vi "UnscentedKalmanFilter_SetXHat_Single.vi"(9 "xHat Value":dbl, 10 "Row":i32, 11 "in UnscentedKalmanFiilter":T1) -> (3 "out UnscentedKalmanFiilter":T1)   [LabVIEW 2019, in "Trajectory_Library.lvlib"]
doc: "Creates a new LINEAR SYSTEM data cluster with the specified values. \n\n\nInputs: \n - XXX -- XXX.\n\nOutputs:\n - XXX -- XXX."
uses:
  Trajectory_Library.lvlib
  <vilib>/Analysis/Matrix/Datatypes/RealMatrix.ctl
  <vilib>/Analysis/Matrix/NI_Matrix.lvlib
  MERWE_SCALED_SIGMA_PTS.ctl
  UNSCENTED_KALMAN_FILTER.ctl
  BiFun_Matrix_FUNC_TYPE.ctl
panel:
  # "State Estimate <Statess,1>"
  # "<States, States>"
  # "<States, ?>"
  # "<Statess,  States>"
  # "<Outputs, Outputs>"
  # "<?, 1>"
  # "<?, 1>"
  # "State Estimate <Statess,1>"
  # "<States, States>"
  # "<States, ?>"
  # "<Statess,  States>"
  # "<Outputs, Outputs>"
  # "<?, 1>"
  # "<?, 1>"
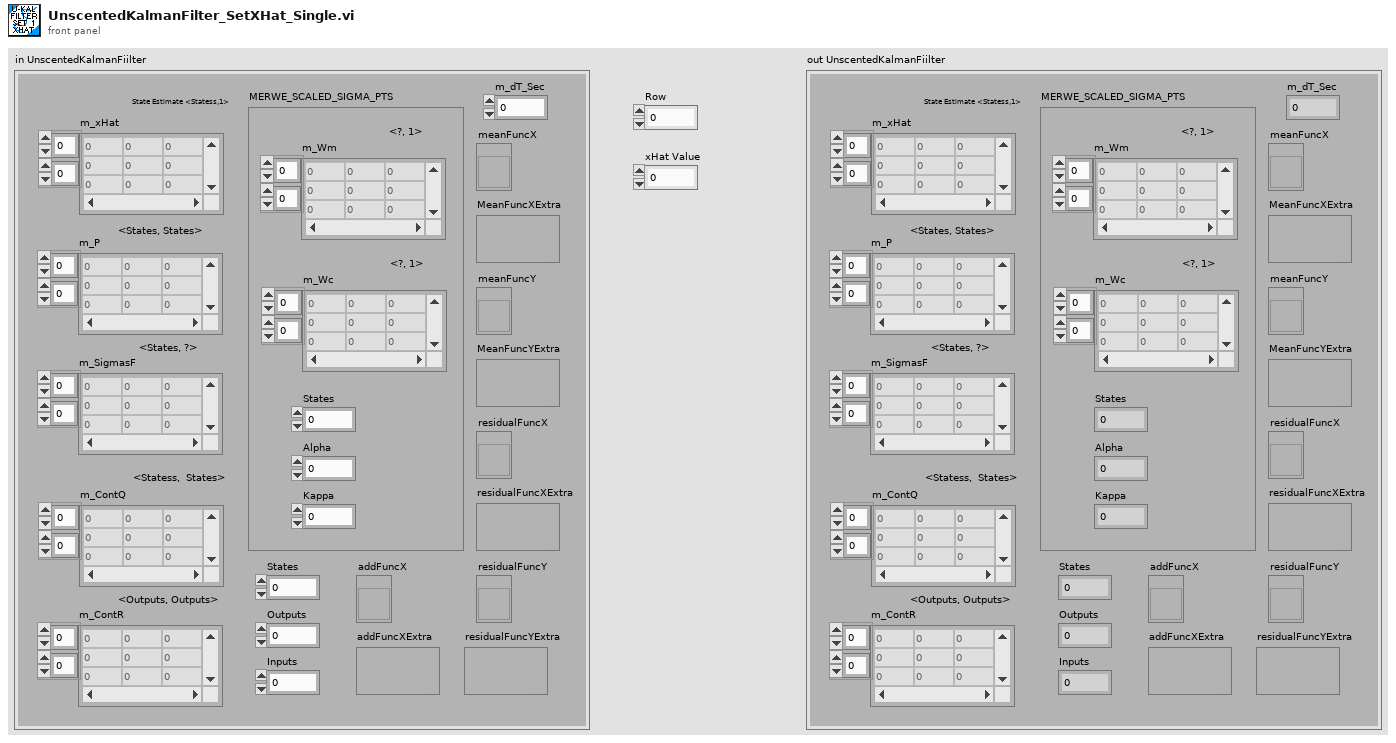
[diagram p1: front panel]
types:
  T1 = typedef "Trajectory_Library.lvlib/UNSCENTED_KALMAN_FILTER.ctl" = cluster{"m_P":T2, "m_xHat":T2, "States":i32, "Outputs":i32, "m_ContR":T2, "m_ContQ":T2, "m_SigmasF":T2, "m_dT_Sec":dbl, "MERWE_SCALED_SIGMA_PTS":T3, "meanFuncX":T4, "meanFuncY":T4, "residualFuncX":T4, "residualFuncY":T4, "addFuncX":T4, "addFuncXExtra":variant, "residualFuncYExtra":variant, "residualFuncXExtra":variant, "MeanFuncYExtra":variant, "MeanFuncXExtra":variant, "Inputs":i32}
  T2 = typedef "NI_Matrix.lvlib/RealMatrix.ctl" = dbl[][]
  T3 = typedef "Trajectory_Library.lvlib/MERWE_SCALED_SIGMA_PTS.ctl" = cluster{"m_Wm":T2, "States":i32, "Alpha":dbl, "m_Wc":T2, "Kappa":i32}
  T4 = typedef "Trajectory_Library.lvlib/BiFun_Matrix_FUNC_TYPE.ctl" = refnum<vi>
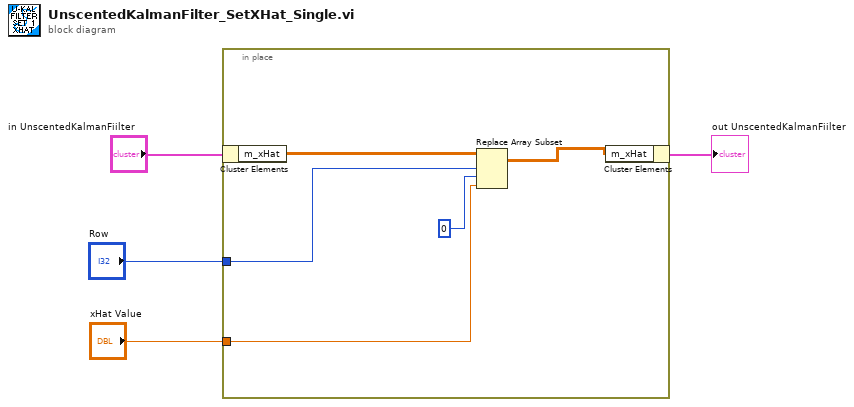
[diagram p0: block diagram]
diagram:
  n1 = in-place {
    in-place-border: "Row" -> [w6]
    in-place-border: "xHat Value" -> [w5]
    n2 = in-place-cluster #1("in UnscentedKalmanFiilter") -> ("m_xHat"=w9:T2)
    n3 = Replace Array Subset(array=w9, new element=w5, index (row)=w6, index (col)=0) -> (w8:T2)
    n4 = in-place-cluster #1("m_xHat"=w8) -> (→"out UnscentedKalmanFiilter":T1)
  }
